vi "Refresh Signals Compare To Existing.vi"(8 "error in":errorcluster, 10 "Database Signals":T2[](array[typedef]), 11 "Frame Sysdef":T1 format="%.0x") -> (0 "error out":errorcluster, 2 "Unmatched Signals":T2[](array[typedef]), 3 "Refresh Signals":T3[](array[typedef]))   [LabVIEW 2020, in "Communication Bus Template System Explorer.lvlib" / "Implementation.lvlib"]
uses:
  Types/Signal.ctl
  Types/Refresh Signal.ctl
  <vilib>/NI VeriStand/Custom Device API/Custom Device Item Ref.ctl
  Implementation.lvlib
  Scripting/Communication Bus Template Scripting.lvlib
  <vilib>/NI VeriStand/Custom Device API/Custom Device API.lvlib
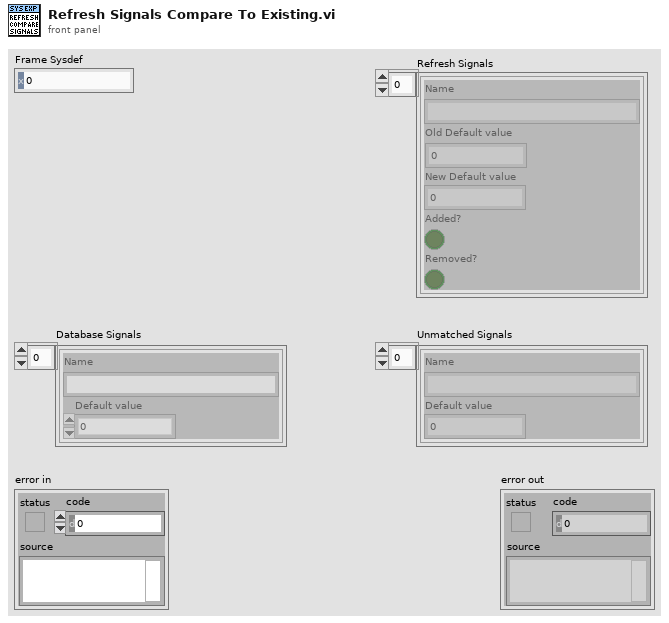
[diagram p1: front panel]
types:
  T1 = typedef "Custom Device API.lvlib/Custom Device Item Ref.ctl" = u64
  T2 = typedef "Communication Bus Template System Explorer.lvlib/Implementation.lvlib/Signal.ctl" = cluster{"Name":string, "Default value":dbl}
  T3 = typedef "Communication Bus Template System Explorer.lvlib/Implementation.lvlib/Refresh Signal.ctl" = cluster{"Name":string, "Old Default value":dbl, "New Default value":dbl, "Added?":bool, "Removed?":bool}
  T4 = typedef "Custom Device API.lvlib/Custom Device Channel.ctl" = cluster{"Type":T5, "Units":string, "Default Value":dbl, "Faultable":bool, "Scalable":bool}
  T5 = typedef "Custom Device API.lvlib/Custom Device Channel Type.ctl" = enum16{"Input", "Output"}
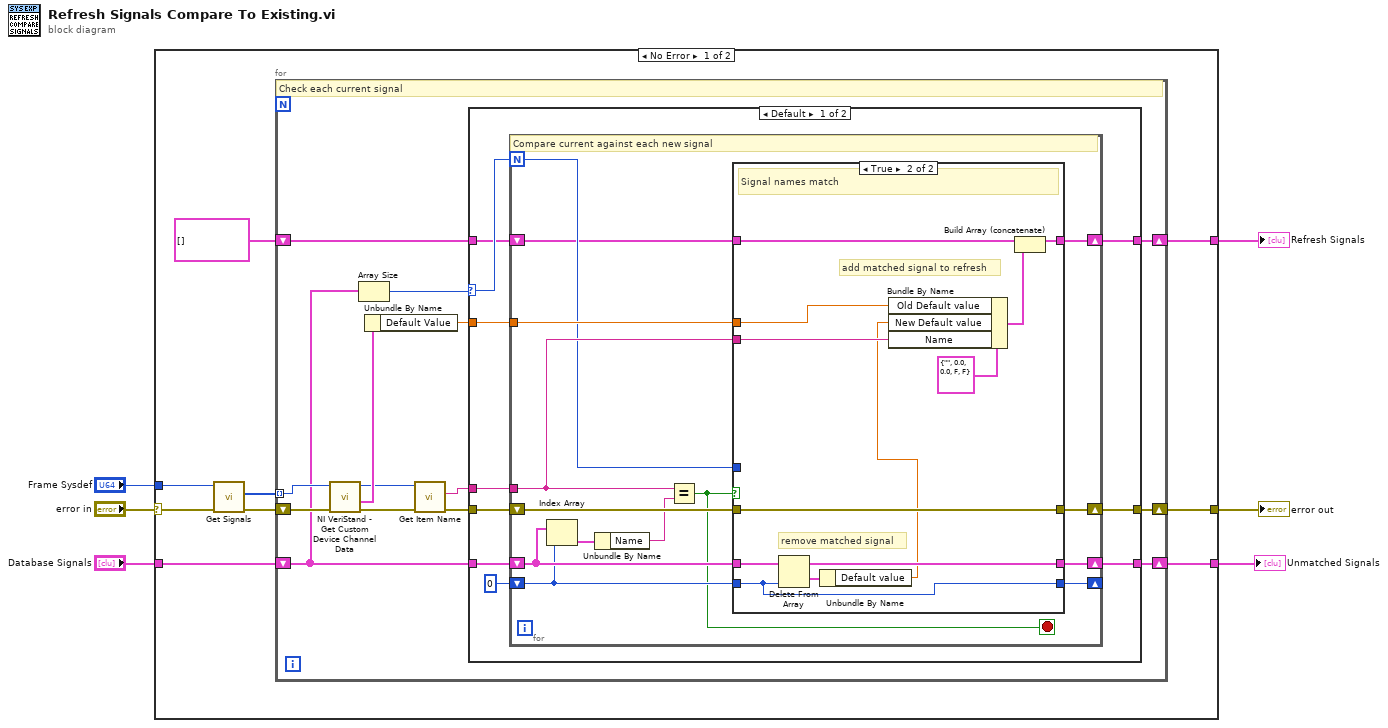
[diagram p0: block diagram]
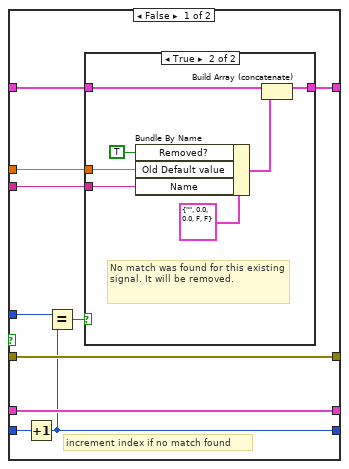
[diagram p2: hidden frame]
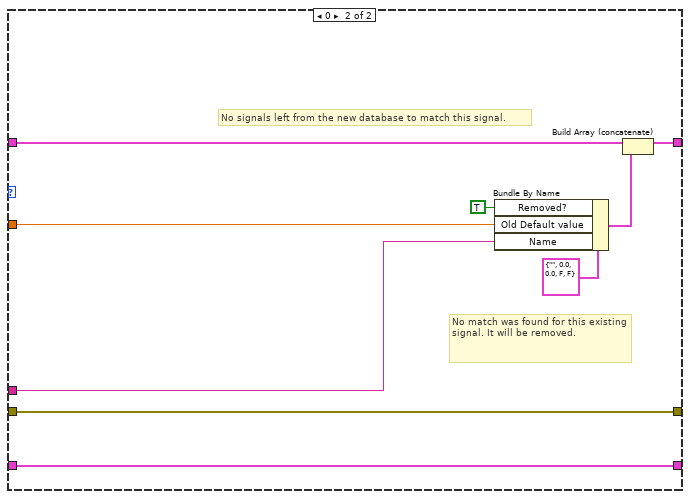
[diagram p4: hidden frame]
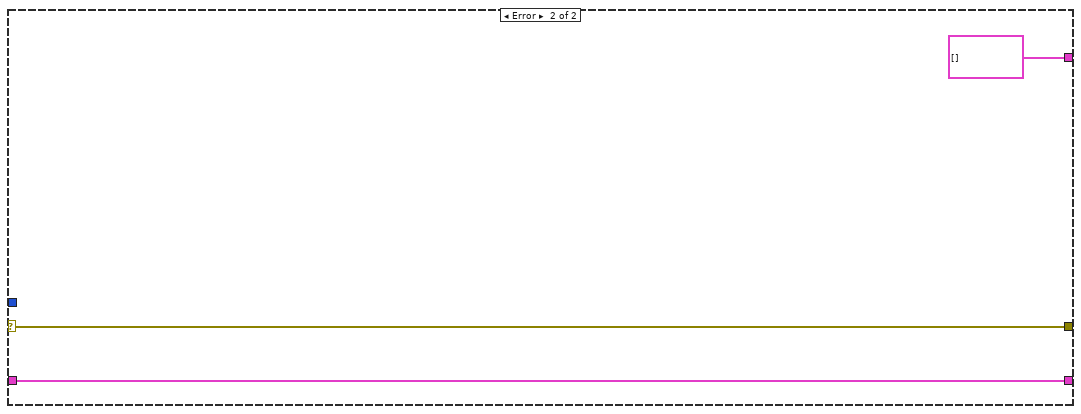
[diagram p5: hidden frame]
diagram:
  n1 = case shown="No Error" "error in" {
    selector: "error in" -> [w9 w95]
    tunnel: [w8 w95] -> w5
    tunnel: "Database Signals" -> [w12 w93]
    tunnel: [w11 T3[] [] ("Refresh Signals")] -> w3
    tunnel: [w10 w93] -> w2
    tunnel: "Frame Sysdef" -> [w7 _]
    frame No Error {
      n2 = call "Get Signals.vi"("error in"=w9, "Frame in"=w7) -> ("error out"=w15:errorcluster, "Signals"=w14:T1[])  [unwired: 7 in, 1 out]
      n3 = for {
        tunnel: w14 -> [w28] mode=indexing
        shift-right: [w19] -> w10
        shift-left: w12 -> [w22]
        shift-right: [w20] -> w8
        shift-left: w15 -> [w29]
        shift-right: [w16] -> w11
        shift-left: T3[] [] ("Refresh Signals") -> [w17]
        # "Check each current signal"
        n4 = call <vilib>:"NI VeriStand - Get Custom Device Channel Data.vi"("error in (no error)"=w29, "Channel Ref in"=w28) -> ("error out"=w25:errorcluster, "Channel"=w27:T4, "Channel Ref out"=w26:T1)  [unwired: 4 in, 3 out]
        n5 = Array Size(array=w22) -> (size(s)=w18:i32)
        n6 = Unbundle By Name(w27) -> ("Default Value"=w21:dbl)
        n7 = call "Get Item Name.vi"("error in"=w25, "Item Ref"=w26) -> ("error out"=w24:errorcluster, "Name"=w23:string)  [unwired: 7 in, 1 out]
        n8 = case shown="Default" w18 {
          selector: w18 -> [w32 _]
          tunnel: w24 -> [w39 w92]
          tunnel: w23 -> [w38 w86]
          tunnel: w22 -> [w36 w91]
          tunnel: w21 -> [w35 w85]
          tunnel: [w34 w92] -> w20
          tunnel: [w33 w91] -> w19
          tunnel: w17 -> [w31 w87]
          tunnel: [w30 w84] -> w16
          frame Default {
            n9 = for {
              N: w32 -> [w42]
              shift-right: [w47] -> w33
              shift-left: w36 -> [w50]
              shift-right: [w43] -> w34
              shift-left: w39 -> [w53]
              tunnel: w38 -> [w46]
              shift-right: [w48] -> _
              shift-left: 0 -> [w49]
              tunnel: w35 -> [w44]
              shift-right: [w40] -> w30
              shift-left: w31 -> [w41]
              stop <- w45 stop-if-true
              # "Compare current against each new signal"
              n10 = Index Array(array=w50, index=w49) -> (element=w52:T2)
              n11 = Unbundle By Name(w52) -> ("Name"=w51:string)
              n12 = Equal?(x=w46, y=w51) -> (x = y?=w45:bool)
              n13 = case shown="True" w45 {
                tunnel: w53 -> [w60 w79]
                tunnel: w50 -> [w63 w83]
                tunnel: w49 -> [w56 w82]
                tunnel: [w57 w82] -> w48
                tunnel: [w63 w81] -> w47
                tunnel: w46 -> [w58 w74]
                tunnel: w44 -> [w61 w72]
                tunnel: w42 -> [w59 _]
                tunnel: [w60 w79] -> w43
                tunnel: w41 -> [w55 w75]
                tunnel: [w54 w76] -> w40
                frame False {
                  # "increment index if no match found"
                  n14 = Increment(x=w56) -> (x+1=w57:i32)
                  n15 = Equal?(x=w59, y=w57) -> (x = y?=w62:bool)
                  n16 = case shown="True" w62 {
                    tunnel: w58 -> [_ w68]
                    tunnel: w61 -> [_ w67]
                    tunnel: w55 -> [w64 w71]
                    tunnel: [w64 w70] -> w54
                    frame False {
                    }
                    frame True {
                      # "No match was found for this existing signal. It will be removed."
                      n17 = Bundle By Name(cluster=T3 {"Name"="", "Old Default value"=0.0, "New Default value"=0.0, "Added?"=FALSE, "Removed?"=FALSE} ("Refresh Signal"), "Removed?"=TRUE, "Old Default value"=w67, "Name"=w68) -> (w65:T3)
                      n18 = Build Array (concatenate)(w71, w65) -> (w70:T3[])
                    }
                  }
                }
                frame True {
                  # "add matched signal to refresh"
                  # "remove matched signal"
                  # "Signal names match"
                  n19 = Delete From Array(array=w83, index=w82) -> (deleted portion=w80:T2, array with subset deleted=w81:T2[])  [unwired: 1 in]
                  n20 = Unbundle By Name(w80) -> ("Default value"=w73:dbl)
                  n21 = Bundle By Name(cluster=T3 {"Name"="", "Old Default value"=0.0, "New Default value"=0.0, "Added?"=FALSE, "Removed?"=FALSE} ("Refresh Signal"), "Old Default value"=w72, "New Default value"=w73, "Name"=w74) -> (w77:T3)
                  n22 = Build Array (concatenate)(w75, w77) -> (w76:T3[])
                }
              }
            }
          }
          frame 0 {
            # "No signals left from the new database to match this signal."
            # "No match was found for this existing signal. It will be removed."
            n23 = Bundle By Name(cluster=T3 {"Name"="", "Old Default value"=0.0, "New Default value"=0.0, "Added?"=FALSE, "Removed?"=FALSE} ("Refresh Signal"), "Removed?"=TRUE, "Old Default value"=w85, "Name"=w86) -> (w88:T3)
            n24 = Build Array (concatenate)(w87, w88) -> (w84:T3[])
          }
        }
      }
    }
    frame Error {
    }
  }
  "error out" <- w5
  "Refresh Signals" <- w3
  "Unmatched Signals" <- w2
